vi "ReadID.vi"(8 "ErrorIn":errorcluster, 11 "ReferenceIn":refnum<class "JSONTextViewer.lvclass">) -> (0 "ErrorOut":errorcluster, 2 "ID":string, 3 "ReferenceIn":refnum<class "JSONTextViewer.lvclass">)   [LabVIEW 2021, in "JSONTextViewer.lvlib" / "JSONTextViewer.lvclass"]
uses:
  JSONTextViewer.lvclass
  JSONTextViewer.lvclass/JSONTextViewer.ctl
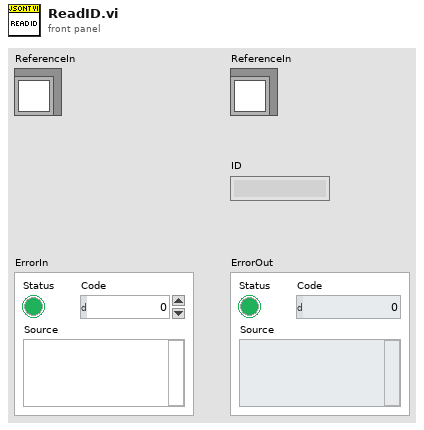
[diagram p1: front panel]
types:
  T1 = typedef "JSONTextViewer.lvlib/JSONTextViewer.lvclass/ObjectAttributes.ctl" = cluster{"Interfaces":cluster{"ApplicationConfiguration":refnum<class "IApplicationConfiguration.lvclass">}, "Locals":cluster{"MainGUIActive":refnum<queue>, "JSONText":string, "ID":string}, "Persistent":cluster{"Dummy":bool}}
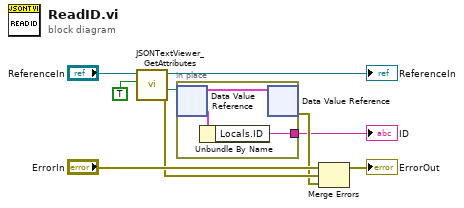
[diagram p0: block diagram]
diagram:
  n1 = call "JSONTextViewer_GetAttributes.vi"("OnlyGetDvrReference(False)"=TRUE, "ReferenceIn"="ReferenceIn") -> ("ErrorOut"=w8:errorcluster, "DataRef"=w2:refnum<data-value>, "ReferenceOut"=→"ReferenceIn":refnum<class "JSONTextViewer.lvclass">)  [unwired: 6 in, 1 out]
  n2 = in-place {
    in-place-border: [w11] -> w1
    n3 = in-place-dvr #1(w2) -> (w10:T1)  [unwired: 1 out]
    n4 = Unbundle By Name(w10) -> ("Locals.ID"=w11:string)
    n5 = in-place-dvr #1(w10) -> (w6:errorcluster)  [unwired: 1 out]
  }
  "ID" <- w1
  n6 = Merge Errors("ErrorIn", w8, w6) -> (→"ErrorOut":errorcluster)
